vi "PositionTactic.vi"(0 "object in":refnum<class "PositionTactic.lvclass">, 5 "error in (no error)":errorcluster) -> (14 "object out":refnum<class "PositionTactic.lvclass">, 19 "error out":errorcluster)   [LabVIEW 2023, in "PositionTactic.lvclass"]
uses:
  PositionTactic.lvclass
  PositionTactic.lvclass/PositionTactic.ctl
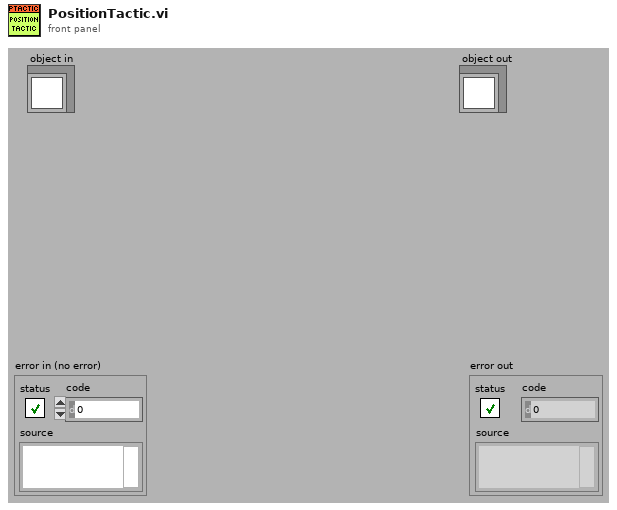
[diagram p1: front panel]
types:
  T1 = typedef "PositionTactic.lvclass/PositionTactic_states.ctl" = enum16{"GoToGuardPosition\n", "GoToTarget\n", "Exit"}
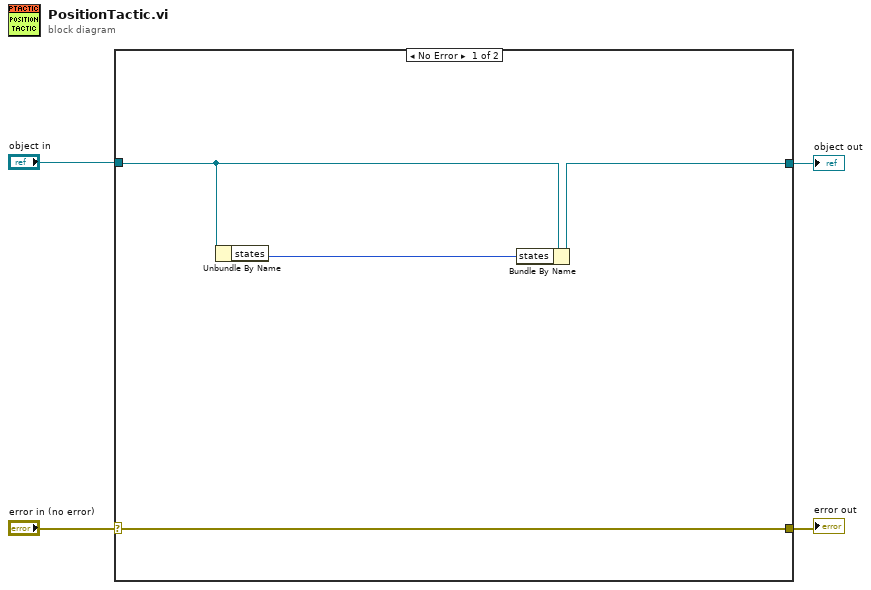
[diagram p0: block diagram]
diagram:
  n1 = case shown="No Error" "error in (no error)" {
    selector: "error in (no error)" -> [w7 w10]
    tunnel: [w7 w10] -> w3
    tunnel: [w5 w9] -> w1
    tunnel: "object in" -> [w6 w9]
    frame No Error {
      n2 = Unbundle By Name(w6) -> ("states"=w8:T1)
      n3 = Bundle By Name(cluster=w6, "states"=w8) -> (w5:refnum<class "PositionTactic.lvclass">)
    }
    frame Error {
    }
  }
  "error out" <- w3
  "object out" <- w1
